vi "SMR_LabVIEW_V7.vi"() -> ()   [LabVIEW 2025]
uses:
  <vilib>/DAQmx/write.llb/DAQmx Write (Analog DBL 1Chan 1Samp).vi
  <vilib>/DAQmx/read.llb/DAQmx Read (Analog 1D DBL NChan 1Samp).vi
  <vilib>/DAQmx/create/channels.llb/DAQmx Create Channel (AI-Temperature-Thermocouple).vi
  <vilib>/DAQmx/create/channels.llb/DAQmx Create Channel (AI-Voltage-Basic).vi
  <vilib>/DAQmx/create/channels.llb/DAQmx Create Channel (AO-Voltage-Basic).vi
  <vilib>/DAQmx/miscellaneous.llb/DAQmx Fill In Error Info.vi
panel:
  in  "P-Valve Command Voltage (V)":dbl min=0.0 max=10.0
  out "Rate Window Ready":bool
  out "Steady State":bool
  in  "Steady State Threshold (deg C/min)":dbl=0.5
  out "Temp Change Rate (deg C/min)":dbl
  in  "Voltage Limit (V)":dbl=10.0
  in  "Temperature Limit (C)":dbl=50.0
  in  "Pressure Limit (psi)":dbl=15.0
  out "Max Voltage":bool
  out "Max Temperature":bool
  out "Max Pressure":bool
  out "Current Run Folder":path
  in  "Log Root Folder":path=path "C:/Users/LocalUser/Documents/GitHub/thermal-loop/resources/v0.1.1/data/001"
  out "Heat Exchanger Pressure History":dbl(graph)
  out "Main Loop Pressure History":T1(graph)
  out "Heat Exchanger Temperature History":cluster{"Waveform":dbl, "Waveform":dbl}(graph)
  out "Main Loop Temeperature History":T2(graph)
  out "Overall Avg Pressure (psi)":dbl
  out "Heat Exchanger Pressure P6 (psi)":dbl
  out "Main Loop Avg Pressure (psi)":dbl
  out "Heat Exchanger Avg Temp (deg C)":dbl
  out "Main Loop Avg Temp (deg C)":dbl
  out "Raw NI9201 \nVoltage Display":T3
  out "Temperature Display":T4
  out "Pressure Display":T5
  in  "Flow Offset Correction (GPM)":dbl=-0.3
  out "Flow History":dbl(graph)
  out "Overall Pressure History":T6(graph)
  out "Overall Temperature History":T7(graph)
  out "Max Loop Pressure (psi)":dbl
  out "Overall Avg Temp (deg C)":dbl
  out "Max Loop Temp (deg C)":dbl
  out "Heat Exchanger Flow (GPM)":dbl
  in  "Loop Period (ms)":dbl=1000.0
  in  "Stop":bool
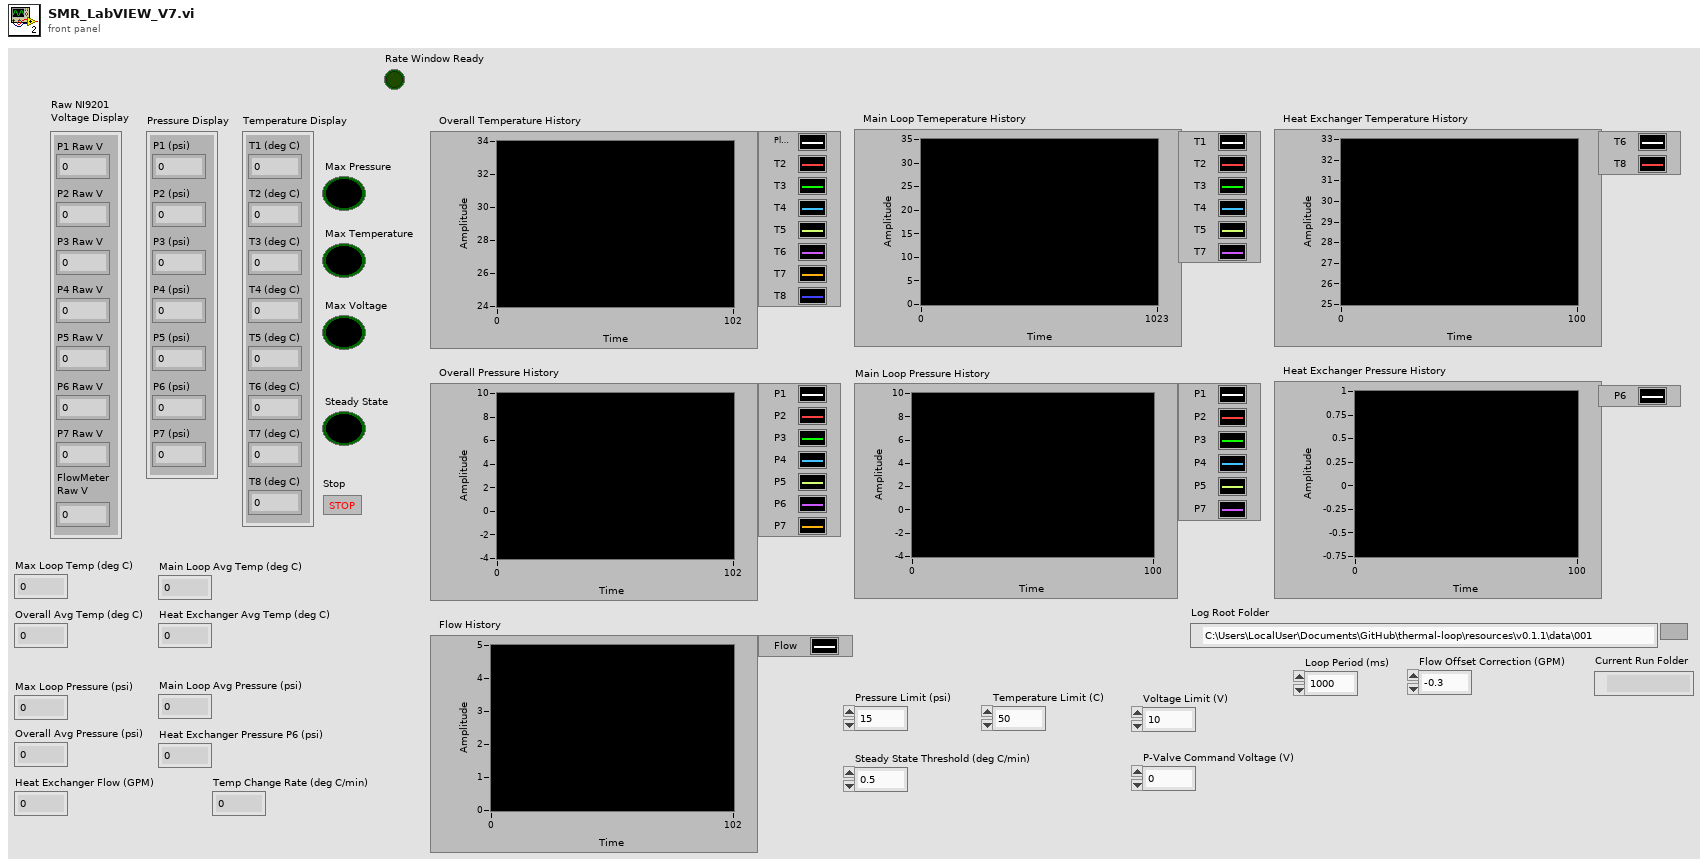
[diagram p1: front panel]
types:
  T1 = cluster{"P1":dbl, "P2":dbl, "P3":dbl, "P4":dbl, "P5":dbl, "P7":dbl}
  T2 = cluster{"Waveform":dbl, "Waveform":dbl, "Waveform":dbl, "Waveform":dbl, "Waveform":dbl, "Waveform":dbl}
  T3 = cluster{"P1 Raw V":dbl, "P2 Raw V":dbl, "P3 Raw V":dbl, "P4 Raw V":dbl, "P5 Raw V":dbl, "P6 Raw V":dbl, "P7 Raw V":dbl, "FlowMeter\nRaw V":dbl}
  T4 = cluster{"T1 (deg C)":dbl, "T2 (deg C)":dbl, "T3 (deg C)":dbl, "T4 (deg C)":dbl, "T5 (deg C)":dbl, "T6 (deg C)":dbl, "T7 (deg C)":dbl, "T8 (deg C)":dbl}
  T5 = cluster{"P1 (psi)":dbl, "P2 (psi)":dbl, "P3 (psi)":dbl, "P4 (psi)":dbl, "P5 (psi)":dbl, "P6 (psi)":dbl, "P7 (psi)":dbl}
  T6 = cluster{"P1":dbl, "P2":dbl, "P3":dbl, "P4":dbl, "P5":dbl, "P6":dbl, "P7":dbl}
  T7 = cluster{"Waveform":dbl, "Waveform":dbl, "Waveform":dbl, "Waveform":dbl, "Waveform":dbl, "Waveform":dbl, "Waveform":dbl, "Waveform":dbl}
  T8 = enum16{"open", "replace", "create", "open or create", "replace or create", "replace or create with confirmation"}
  T9 = cluster{"P1":dbl, "P2":dbl, "P3":dbl, "P4":dbl, "P5":dbl, "P6":dbl, "P7":dbl, "Flow":dbl}
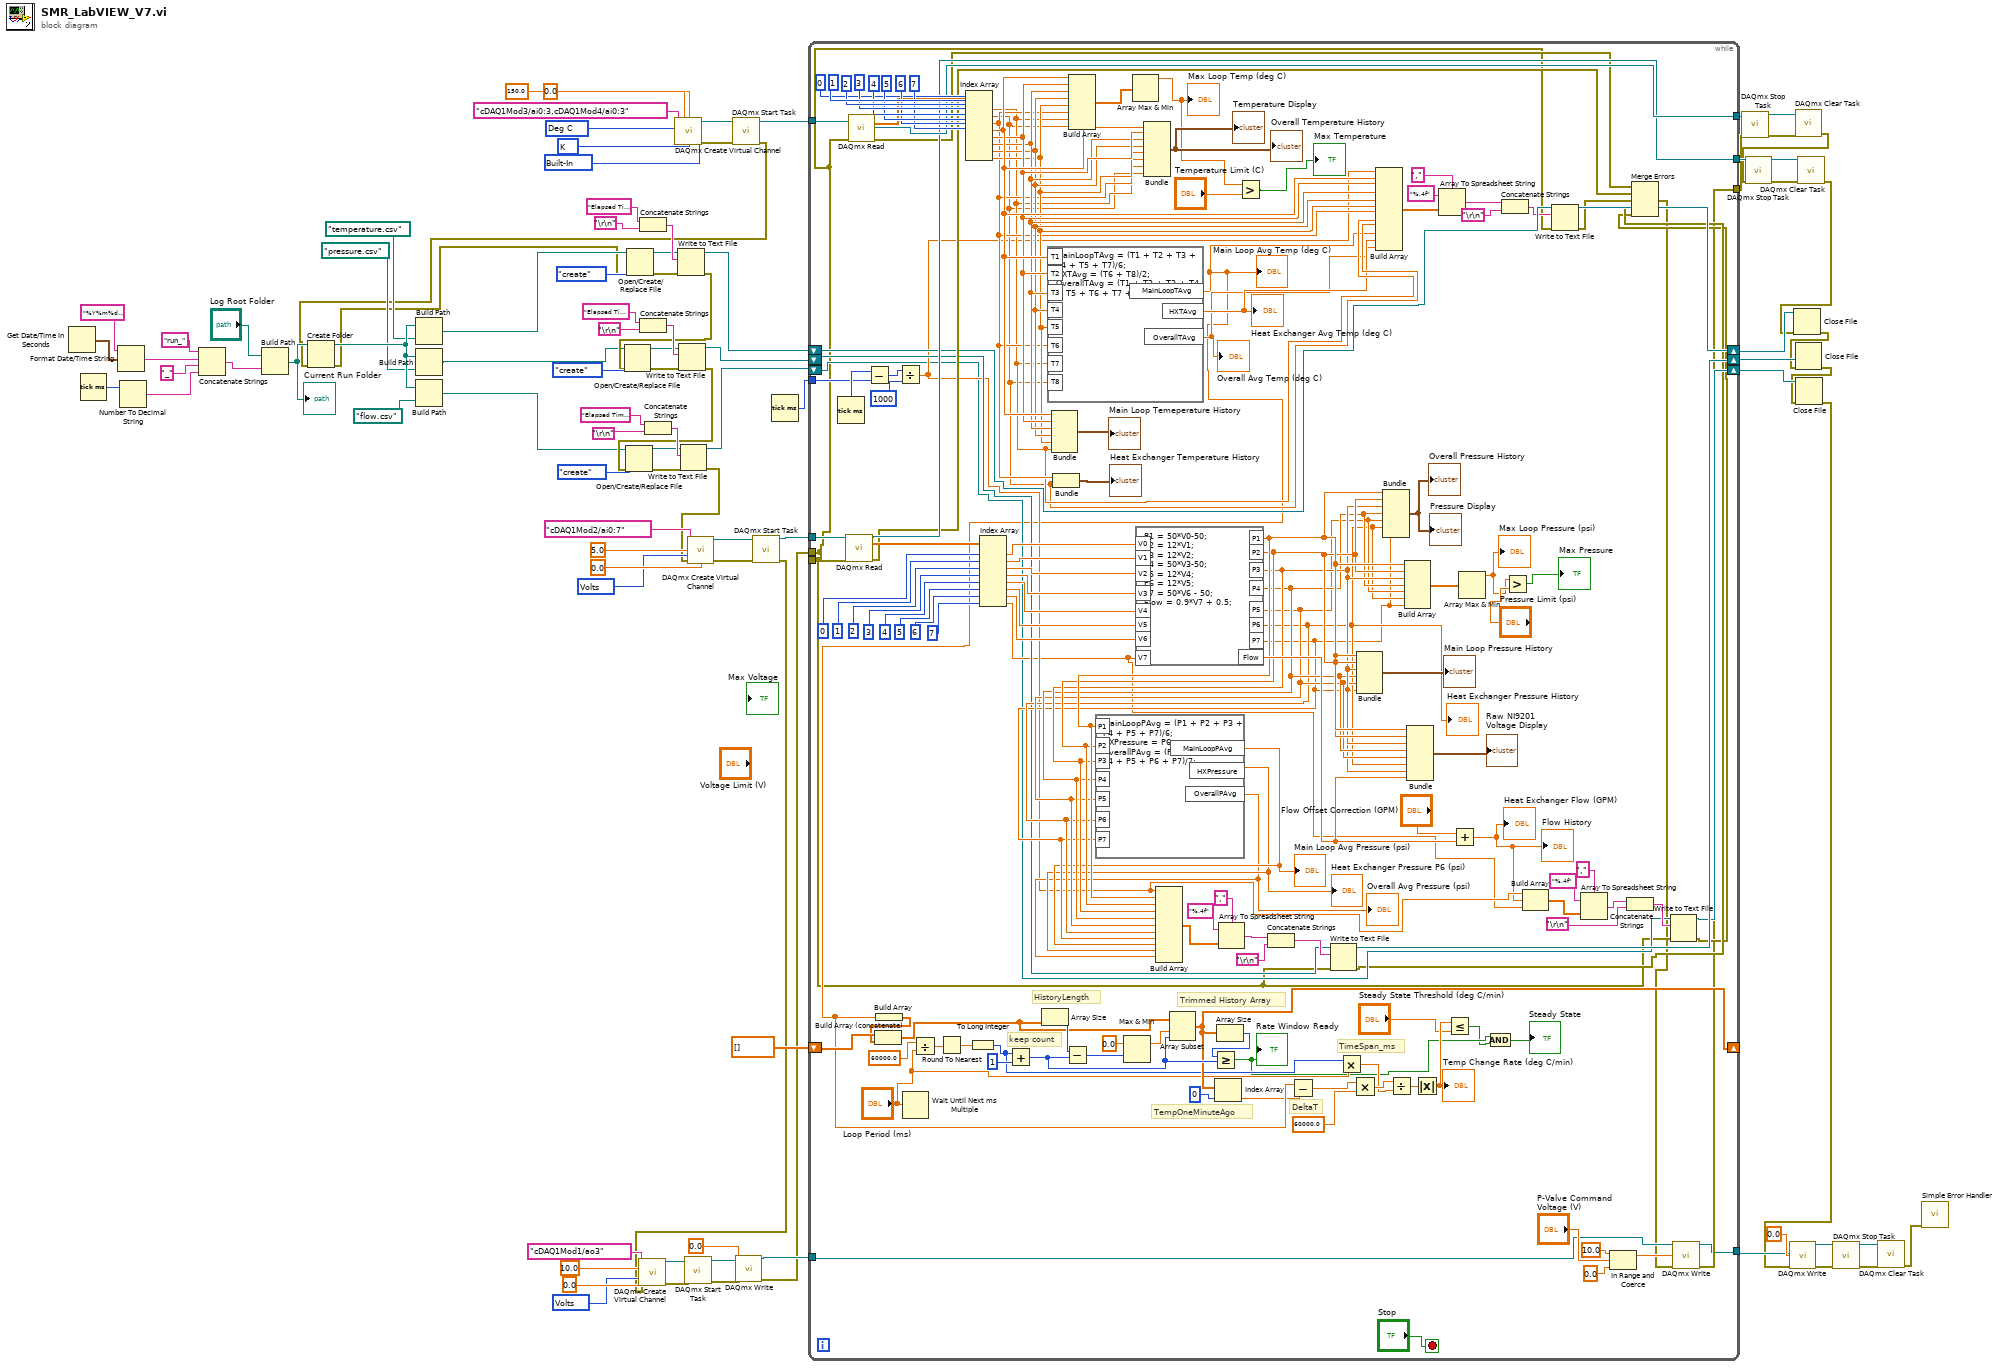
[diagram p0: block diagram]
diagram:
  w17 = 10348 items=["Volts"=10348, "From Custom Scale"=10065] ("units")
  w83 = 10200 items=["Built-In"=10200, "Constant Value"=10116, "Channel"=10113] ("cjc source")
  w84 = 10073 items=["J"=10072, "K"=10073, "N"=10077, "R"=10082, "S"=10085, "T"=10086, "B"=10047, "E"=10055] ("thermocouple type")
  w85 = 10143 items=["Deg C"=10143, "Deg F"=10144, "Kelvins"=10325, "Deg R"=10145, "From Custom Scale"=10065] ("units")
  w92 = 10348 items=["Volts"=10348, "From Custom Scale"=10065] ("units")
  n1 = Get Date/Time In Seconds() -> (seconds since 1Jan1904=w40:timestamp)
  n2 = Tick Count (ms)() -> (millisecond timer value=w38:u32)
  n3 = Format Date/Time String(time format string (%c)="%Y%m%d_%H%M%S", seconds (now)=w40) -> (date/time string=w35:string)  [unwired: 1 in]
  n4 = Number To Decimal String(number=w38) -> (decimal integer string=w36:string)  [unwired: 1 in]
  n5 = Concatenate Strings("run_" ("string"), w35, "_" ("string"), w36) -> (w32:string)
  n6 = Build Path(base path="Log Root Folder", name or relative path=w32) -> (appended path=w31:path)
  "Current Run Folder" <- w31
  n7 = Concatenate Strings("Elapsed Time (s),T1 (deg C),T2 (deg C),T3 (deg C),T4 (deg C),T5 (deg C),T6 (deg C),T7 (deg C),T8 (deg C),Main Loop Avg Temp (deg C),HX Avg Temp (deg C),Overall Avg Temp (deg C)", "\r\n") -> (w66:string)
  n8 = Concatenate Strings("Elapsed Time (s),P1 (psi),P2 (psi),P3 (psi),P4 (psi),P5 (psi),P6 (psi),P7 (psi),Main Loop Avg Pressure (psi),HX Pressure (psi),Overall Avg Pressure (psi)", "\r\n") -> (w64:string)
  n9 = Concatenate Strings("Elapsed Time (s),Heat Exchanger Flow (GPM),Flow Raw Voltage (V)", "\r\n") -> (w60:string)
  n10 = call-poly <vilib>:"DAQmx Create Virtual Channel.vi"("maximum value"=150.0, "minimum value"=0.0, "physical channels"=tag "cDAQ1Mod3/ai0:3,cDAQ1Mod4/ai0:3", "cjc source"=w83, "units"=w85, "thermocouple type"=w84) -> ("task out"=w82:refnum<k21>, "error out"=w81:errorcluster)  [unwired: 8 in]
  n11 = call <vilib>:"DAQmx Start Task.vi"("task/channels in"=w82, "error in"=w81) -> ("task out"=w80:refnum<k21>, "error out"=w23:errorcluster)  [unwired: 12 in]
  n12 = Create Folder(path (use dialog)=w31, error in=w23) -> (created path=w30:path, error out=w22:errorcluster)  [unwired: 1 in, 1 out]
  n13 = Build Path(base path=w30, name or relative path=path "temperature.csv") -> (appended path=w29:path)
  n14 = Build Path(base path=w30, name or relative path=path "pressure.csv") -> (appended path=w28:path)
  n15 = Build Path(base path=w30, name or relative path=path "flow.csv") -> (appended path=w27:path)
  n16 = Open/Create/Replace File(file path (use dialog)=w29, error in=w22, operation (0:open)=T8."create") -> (refnum out=w65:refnum<file>, error out=w49:errorcluster)  [unwired: 3 in, 1 out]
  n17 = Write to Text File(file (use dialog)=w65, text=w66, error in=w49) -> (refnum out=w56:refnum<file>, error out=w48:errorcluster)  [unwired: 1 in, 1 out]
  n18 = Open/Create/Replace File(file path (use dialog)=w28, error in=w48, operation (0:open)=T8."create") -> (refnum out=w63:refnum<file>, error out=w47:errorcluster)  [unwired: 3 in, 1 out]
  n19 = Write to Text File(file (use dialog)=w63, text=w64, error in=w47) -> (refnum out=w55:refnum<file>, error out=w46:errorcluster)  [unwired: 1 in, 1 out]
  n20 = Open/Create/Replace File(file path (use dialog)=w27, error in=w46, operation (0:open)=T8."create") -> (refnum out=w59:refnum<file>, error out=w45:errorcluster)  [unwired: 3 in, 1 out]
  n21 = Write to Text File(file (use dialog)=w59, text=w60, error in=w45) -> (refnum out=w54:refnum<file>, error out=w44:errorcluster)  [unwired: 1 in, 1 out]
  n22 = call-poly <vilib>:"DAQmx Create Virtual Channel.vi"("maximum value"=5.0, "minimum value"=0.0, "physical channels"=tag "cDAQ1Mod2/ai0:7", "units"=w92, "error in"=w44) -> ("task out"=w91:refnum<k21>, "error out"=w90:errorcluster)  [unwired: 9 in]
  n23 = call <vilib>:"DAQmx Start Task.vi"("task/channels in"=w91, "error in"=w90) -> ("task out"=w89:refnum<k21>, "error out"=w10:errorcluster)  [unwired: 12 in]
  n24 = call-poly <vilib>:"DAQmx Create Virtual Channel.vi"("maximum value"=10.0, "minimum value"=0.0, "physical channels"=tag "cDAQ1Mod1/ao3", "units"=w17, "error in"=w10) -> ("task out"=w16:refnum<k21>, "error out"=w15:errorcluster)  [unwired: 9 in]
  n25 = call <vilib>:"DAQmx Start Task.vi"("task/channels in"=w16, "error in"=w15) -> ("task out"=w14:refnum<k21>, "error out"=w13:errorcluster)  [unwired: 12 in]
  n26 = call-poly <vilib>:"DAQmx Write.vi"("task/channels in"=w14, "data"=0.0, "error in"=w13) -> ("task out"=w11:refnum<k21>, "error out"=w9:errorcluster)  [unwired: 10 in, 1 out]
  n27 = Tick Count (ms)() -> (millisecond timer value=w53:u32)
  n28 = while {
    tunnel: w89 -> [w233]
    tunnel: w80 -> [w207]
    tunnel: [w197] -> w79
    tunnel: [w99] -> _
    tunnel: [w196] -> w78
    tunnel: [w97] -> w77
    shift-right: [w173] -> w52
    shift-left: w56 -> [w174]
    shift-right: [w154] -> w51
    shift-left: w55 -> [w155]
    shift-right: [w143] -> w50
    shift-left: w54 -> [w144]
    tunnel: w53 -> [w192]
    shift-right: [w120] -> _
    shift-left: dbl[] [] -> [w133]
    tunnel: w11 -> [w100]
    tunnel: w9 -> [w99]
    tunnel: [w96] -> w7
    stop <- "Stop" stop-if-true
    # "TimeSpan_ms"
    # "DeltaT"
    # "TempOneMinuteAgo"
    # "Trimmed History Array"
    # "HistoryLength"
    # "keep count"
    n29 = Tick Count (ms)() -> (millisecond timer value=w193:u32)
    n30 = call-poly <vilib>:"DAQmx Read.vi"("task/channels in"=w233, "error in"=w99) -> ("task out"=w196:refnum<k21>, "data"=w224:dbl[], "error out"=w194:errorcluster)  [unwired: 11 in]
    n31 = call-poly <vilib>:"DAQmx Read.vi"("task/channels in"=w207, "error in"=w99) -> ("task out"=w197:refnum<k21>, "data"=w198:dbl[], "error out"=w195:errorcluster)  [unwired: 11 in]
    n32 = Subtract(x=w193, y=w192) -> (x-y=w191:u32)
    n33 = Divide(x=w191, y=u32 1000) -> (x/y=w153:dbl)
    n34 = Wait Until Next ms Multiple(millisecond multiple="Loop Period (ms)") -> ()  [unwired: 1 out]
    n35 = Divide(x=60000.0, y="Loop Period (ms)") -> (x/y=w130:dbl)
    n36 = Round To Nearest(number=w130) -> (nearest integer value=w129:dbl)
    n37 = Index Array(array=w198, index #1=0 ("index"), index #2=1 ("index"), index #3=2 ("index"), index #4=3 ("index"), index #5=4 ("index"), index #6=5 ("index"), index #7=6 ("index"), index #8=7 ("index")) -> (element #1=w183:dbl, element #2=w182:dbl, element #3=w184:dbl, element #4=w189:dbl, element #5=w188:dbl, element #6=w187:dbl, element #7=w186:dbl, element #8=w185:dbl)
    n38 = To Long Integer(number=w129) -> (32bit integer=w116:i32)
    n39 = Index Array(array=w224, index #1=0 ("index"), index #2=1 ("index"), index #3=2 ("index"), index #4=3 ("index"), index #5=4 ("index"), index #6=5 ("index"), index #7=6 ("index"), index #8=7 ("index")) -> (element #1=w223:dbl, element #2=w222:dbl, element #3=w221:dbl, element #4=w220:dbl, element #5=w219:dbl, element #6=w218:dbl, element #7=w217:dbl, element #8=w151:dbl)
    n40 = Add(x=w116, y=1) -> (x+y=w122:i32)
    n41 = formula code="MainLoopTAvg = (T1 + T2 + T3 + T4 + T5 + T7)/6;\nHXTAvg = (T6 + T8)/2;\nOverallTAvg = (T1 + T2 + T3 + T4 + T5 + T6 + T7 + T8)/8;"("T1"=w189, "T2"=w188, "T3"=w187, "T4"=w186, "T5"=w185, "T6"=w184, "T7"=w183, "T8"=w182) -> ("MainLoopTAvg"=w118:dbl, "HXTAvg"=w181:dbl, "OverallTAvg"=w180:dbl)
    "Overall Avg Temp (deg C)" <- w180
    "Main Loop Avg Temp (deg C)" <- w118
    "Heat Exchanger Avg Temp (deg C)" <- w181
    n42 = Build Array(w118) -> (w132:dbl[])
    n43 = Build Array (concatenate)(w133, w132) -> (w124:dbl[])
    n44 = Array Size(array=w124) -> (size(s)=w127:i32)
    n45 = Bundle("Waveform"=w189, "Waveform"=w188, "Waveform"=w187, "Waveform"=w186, "Waveform"=w185, "Waveform"=w183) -> (→"Main Loop Temeperature History":T2)  [unwired: 1 in]
    n46 = Bundle("Waveform"=w184, "Waveform"=w182) -> (→"Heat Exchanger Temperature History":cluster{"Waveform":dbl, "Waveform":dbl})  [unwired: 1 in]
    n47 = Subtract(x=w127, y=w122) -> (x-y=w125:i32)
    n48 = Build Array(w189, w188, w187, w186, w185, w184, w183, w182) -> (w234:dbl[])
    n49 = Max & Min(x=0.0, y=w125) -> (max(x,y)=w123:dbl)  [unwired: 1 out]
    n50 = Array Max & Min(array=w234) -> (max value=w136:dbl)  [unwired: 3 out]
    "Max Loop Temp (deg C)" <- w136
    n51 = formula code="P1 = 50*V0-50;\nP2 = 12*V1;\nP3 = 12*V2;\nP4 = 50*V3-50;\nP5 = 12*V4;\nP6 = 12*V5; \nP7 = 50*V6 - 50;\nFlow = 0.9*V7 + 0.5;"("V0"=w223, "V1"=w222, "V2"=w221, "V3"=w220, "V4"=w219, "V5"=w218, "V6"=w217, "V7"=w151) -> ("P1"=w172:dbl, "P2"=w171:dbl, "P3"=w170:dbl, "P4"=w169:dbl, "P5"=w168:dbl, "P6"=w167:dbl, "P7"=w166:dbl, "Flow"=w212:dbl)
    "Heat Exchanger Pressure History" <- w167
    n52 = formula code="MainLoopPAvg = (P1 + P2 + P3 + P4 + P5 + P7)/6;\nHXPressure = P6;\nOverallPAvg = (P1 + P2 + P3 + P4 + P5 + P6 + P7)/7;"("P1"=w172, "P2"=w171, "P3"=w170, "P4"=w169, "P5"=w168, "P6"=w167, "P7"=w166) -> ("MainLoopPAvg"=w165:dbl, "HXPressure"=w164:dbl, "OverallPAvg"=w163:dbl)
    "Overall Avg Pressure (psi)" <- w163
    "Heat Exchanger Pressure P6 (psi)" <- w164
    "Main Loop Avg Pressure (psi)" <- w165
    n53 = Bundle("Waveform"=w189, "Waveform"=w188, "Waveform"=w187, "Waveform"=w186, "Waveform"=w185, "Waveform"=w184, "Waveform"=w183, "Waveform"=w182) -> (→"Overall Temperature History" →"Temperature Display":T7)  [unwired: 1 in]
    n54 = Build Array(w153, w172, w171, w170, w169, w168, w167, w166, w165, w164, w163) -> (w162:dbl[])
    n55 = Array Subset(array=w124, index=w123, length=w122) -> (w120:dbl[])
    n56 = Index Array(array=w120, index=0) -> (element=w117:dbl)
    n57 = Array Size(array=w120) -> (size(s)=w121:i32)
    n58 = Greater Or Equal?(x=w121, y=w122) -> (x >= y?=w107:bool)
    "Rate Window Ready" <- w107
    n59 = Array To Spreadsheet String(delimiter (Tab)=",", array=w162, 3:"%.4f" ("format string")) -> (spreadsheet string=w158:string)
    n60 = Greater?(x=w136, y="Temperature Limit (C)") -> (0:→"Max Temperature":bool)
    n61 = Concatenate Strings(w158, "\r\n") -> (w156:string)
    n62 = Subtract(x=w118, y=w117) -> (x-y=w114:dbl)
    n63 = Write to Text File(file (use dialog)=w155, text=w156, error in=w99) -> (refnum out=w154:refnum<file>, error out=w141:errorcluster)  [unwired: 1 in, 1 out]
    n64 = Multiply(x=w116, y="Loop Period (ms)") -> (x*y=w111:dbl)
    n65 = Multiply(x=w114, y=60000.0) -> (x*y=w112:dbl)
    n66 = Bundle("P1"=w172, "P2"=w171, "P3"=w170, "P4"=w169, "P5"=w168, "P7"=w166) -> (→"Main Loop Pressure History":T1)  [unwired: 1 in]
    n67 = Build Array(w153, w189, w188, w187, w186, w185, w184, w183, w182, w118, w181, w180) -> (w179:dbl[])
    n68 = Bundle("P1"=w172, "P2"=w171, "P3"=w170, "P4"=w169, "P5"=w168, "P6"=w167, "P7"=w166) -> (→"Overall Pressure History" →"Pressure Display":T6)  [unwired: 1 in]
    n69 = Divide(x=w112, y=w111) -> (x/y=w110:dbl)
    n70 = Build Array(w172, w171, w170, w169, w168, w167, w166) -> (w215:dbl[])
    n71 = Bundle("P1"=w172, "P2"=w171, "P3"=w170, "P4"=w169, "P5"=w168, "P6"=w167, "P7"=w166, "Flow"=w212) -> (→"Raw NI9201 \nVoltage Display":T9)  [unwired: 1 in]
    n72 = Absolute Value(x=w110) -> (abs(x)=w109:dbl)
    "Temp Change Rate (deg C/min)" <- w109
    n73 = Array To Spreadsheet String(delimiter (Tab)=",", array=w179, 3:"%.4f" ("format string")) -> (spreadsheet string=w176:string)
    n74 = Less Or Equal?(x=w109, y="Steady State Threshold (deg C/min)") -> (x <= y?=w106:bool)
    n75 = Add(x="Flow Offset Correction (GPM)", y=w212) -> (x+y=w152:dbl)
    "Heat Exchanger Flow (GPM)" <- w152
    "Flow History" <- w152
    n76 = Array Max & Min(array=w215) -> (max value=w138:dbl)  [unwired: 3 out]
    "Max Loop Pressure (psi)" <- w138
    n77 = And(x=w107, y=w106) -> (x .and. y?=→"Steady State":bool)
    n78 = Concatenate Strings(w176, "\r\n") -> (w159:string)
    n79 = Greater?(x=w138, y="Pressure Limit (psi)") -> (0:→"Max Pressure":bool)
    n80 = Build Array(w153, w152, w151) -> (w150:dbl[])
    n81 = Write to Text File(file (use dialog)=w174, text=w159, error in=w99) -> (refnum out=w173:refnum<file>, error out=w142:errorcluster)  [unwired: 1 in, 1 out]
    n82 = Array To Spreadsheet String(delimiter (Tab)=",", array=w150, 3:"%.4f" ("format string")) -> (spreadsheet string=w146:string)
    n83 = In Range and Coerce(upper limit=10.0, x="P-Valve Command Voltage (V)", lower limit=0.0) -> (coerced(x)=w101:dbl)  [unwired: 1 out]
    n84 = Concatenate Strings(w146, "\r\n") -> (w145:string)
    n85 = Write to Text File(file (use dialog)=w144, text=w145, error in=w99) -> (refnum out=w143:refnum<file>, error out=w140:errorcluster)  [unwired: 1 in, 1 out]
    n86 = Merge Errors(w195, w194, w142, w141, w140) -> (w98:errorcluster)
    n87 = call-poly <vilib>:"DAQmx Write.vi"("task/channels in"=w100, "data"=w101, "error in"=w98) -> ("task out"=w96:refnum<k21>, "error out"=w97:errorcluster)  [unwired: 10 in, 1 out]
  }
  n88 = call <vilib>:"DAQmx Stop Task.vi"("task/channels in"=w79, "error in"=w77) -> ("task out"=w76:refnum<k21>, "error out"=w74:errorcluster)  [unwired: 12 in]
  n89 = call <vilib>:"DAQmx Clear Task.vi"("task in"=w76, "error in"=w74) -> ("error out"=w73:errorcluster)  [unwired: 13 in]
  n90 = call <vilib>:"DAQmx Stop Task.vi"("task/channels in"=w78, "error in"=w73) -> ("task out"=w75:refnum<k21>, "error out"=w72:errorcluster)  [unwired: 12 in]
  n91 = call <vilib>:"DAQmx Clear Task.vi"("task in"=w75, "error in"=w72) -> ("error out"=w43:errorcluster)  [unwired: 13 in]
  n92 = Close File(refnum=w52, error in=w43) -> (error out=w42:errorcluster)  [unwired: 1 out]
  n93 = Close File(refnum=w51, error in=w42) -> (error out=w41:errorcluster)  [unwired: 1 out]
  n94 = Close File(refnum=w50, error in=w41) -> (error out=w6:errorcluster)  [unwired: 1 out]
  n95 = call-poly <vilib>:"DAQmx Write.vi"("task/channels in"=w7, "data"=0.0, "error in"=w6) -> ("task out"=w5:refnum<k21>, "error out"=w3:errorcluster)  [unwired: 10 in, 1 out]
  n96 = call <vilib>:"DAQmx Stop Task.vi"("task/channels in"=w5, "error in"=w3) -> ("task out"=w4:refnum<k21>, "error out"=w2:errorcluster)  [unwired: 12 in]
  n97 = call <vilib>:"DAQmx Clear Task.vi"("task in"=w4, "error in"=w2) -> ("error out"=w1:errorcluster)  [unwired: 13 in]
  n98 = call <vilib>:"Simple Error Handler.vi"("error in (no error)"=w1) -> ()  [unwired: 4 in, 5 out]
